vi "Setup.vi"(11 "Notifier Transport in":refnum<class "Notifier Transport.lvclass">) -> (0 "Error out":errorcluster, 3 "Notifier Transport out":refnum<class "Notifier Transport.lvclass">)   [LabVIEW 2025, in "jettl.lvlib" / "Transport.lvlib" / "Notifier.lvlib" / "Notifier Transport.lvclass"]
uses:
  Notifier Transport.lvclass
  Notifier Transport.lvclass/Notifier Transport.ctl
  Msg/Msg.lvclass
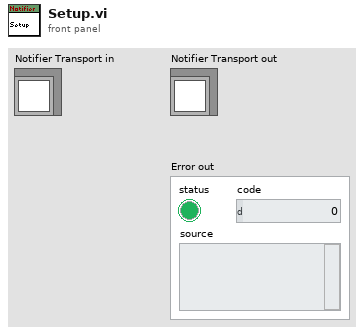
[diagram p1: front panel]
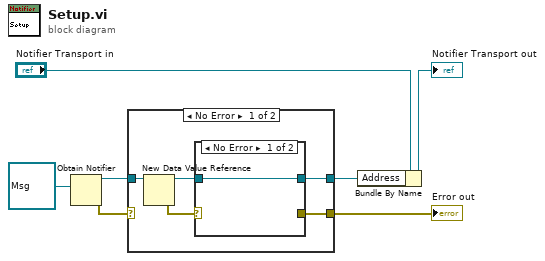
[diagram p0: block diagram]
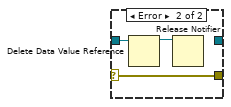
[diagram p2: hidden frame]
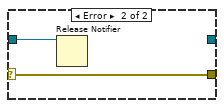
[diagram p3: hidden frame]
diagram:
  n1 = Obtain Notifier(notification data type=refnum<class "Msg.lvclass"> refnum ("Msg")) -> (notifier out=w4:refnum<notifier>, error out=w1:errorcluster)  [unwired: 3 in, 1 out]
  n2 = case shown="No Error" w1 {
    selector: w1 -> [_ w18]
    tunnel: [w10 w18] -> w2
    tunnel: w4 -> [w12 w17]
    tunnel: [w8 _] -> w3
    frame No Error {
      n3 = New Data Value Reference(data value=w12) -> (data value reference=w9:refnum<data-value>, error out=w11:errorcluster)  [unwired: 1 in]
      n4 = case shown="No Error" w11 {
        selector: w11 -> [_ w16]
        tunnel: [_ w16] -> w10
        tunnel: w9 -> [w13 w15]
        tunnel: [w13 _] -> w8
        frame No Error {
        }
        frame Error {
          n5 = Delete Data Value Reference(data value reference=w15) -> (data value=w14:refnum<notifier>)  [unwired: 1 in, 1 out]
          n6 = Release Notifier(notifier=w14) -> ()  [unwired: 2 in, 3 out]
        }
      }
    }
    frame Error {
      n7 = Release Notifier(notifier=w17) -> ()  [unwired: 2 in, 3 out]
    }
  }
  "Error out" <- w2
  n8 = Bundle By Name(cluster="Notifier Transport in", "Address"=w3) -> (→"Notifier Transport out":refnum<class "Notifier Transport.lvclass">)
